vi "jog.vi"() -> ()   [LabVIEW 2018]
uses:
  <vilib>/MediaMongrels Ltd/WebSockets/WebSockets/WebSocket Client/WebSocket Client.lvclass
  D:/software_setup/National Instruments/LabVIEW 2018/vi.lib/MediaMongrels Ltd/WebSockets/WebSockets/WebSocket/WebSocket.lvclass
panel:
  out "GetJOGJointParams_acceleration":dbl[](array[numeric])
  out "GetJOGJointParams_velocity":dbl[](array[numeric])
  out "GetJOGCoordinateParams_acceleration":dbl[](array[numeric])
  out "GetJOGCoordinateParams_velocity":dbl[](array[numeric])
  out "accelerationRatio":i32
  out "velocityRatio":i32
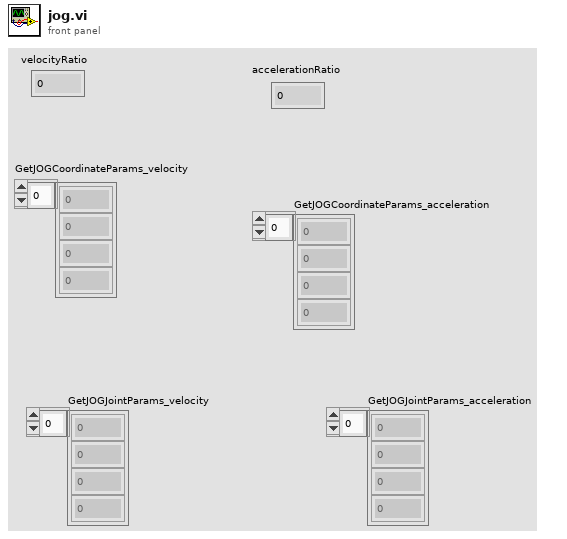
[diagram p1: front panel]
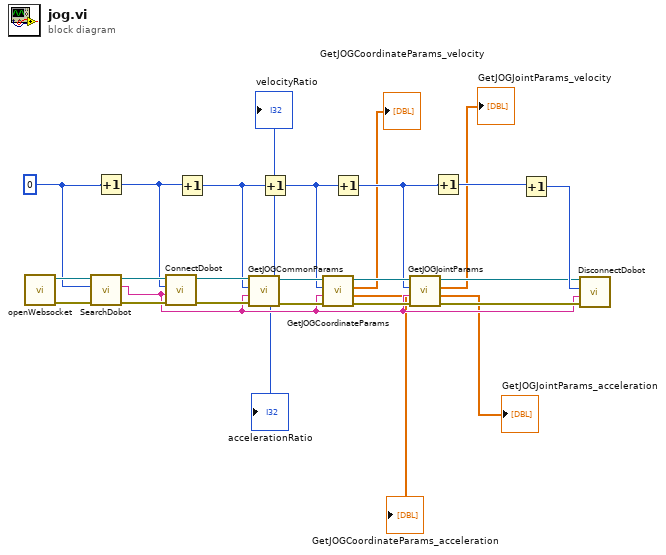
[diagram p0: block diagram]
diagram:
  w22 = 0 ("id")
  n1 = call <vilib>:"openWebsocket.vi"() -> ("error out"=w24:errorcluster, "WebSocket Client out"=w26:refnum<class "WebSocket Client.lvclass">)  [unwired: 10 in]
  n2 = call <vilib>:"SearchDobot.vi"("error in (no error)"=w24, "id"=w22, "WebSocket in"=w26) -> ("error out"=w23:errorcluster, "portName"=w7:string, "WebSocket out"=w25:refnum<class "WebSocket Client.lvclass">)  [unwired: 6 in]
  n3 = Increment(x=w22) -> (x+1=w21:i32)
  n4 = call <vilib>:"ConnectDobot.vi"("error in (no error)"=w23, "portName"=w7, "id"=w21, "WebSocket in"=w25) -> ("error out"=w14:errorcluster, "WebSocket out"=w18:refnum<class "WebSocket Client.lvclass">)  [unwired: 5 in, 1 out]
  n5 = Increment(x=w21) -> (x+1=w10:i32)
  n6 = call <vilib>:"GetJOGCommonParams.vi"("error in (no error)"=w14, "portName"=w7, "id"=w10, "WebSocket in"=w18) -> ("error out"=w13:errorcluster, "accelerationRatio"=→"accelerationRatio":i32, "velocityRatio"=→"velocityRatio":i32, "WebSocket out"=w17:refnum<class "WebSocket Client.lvclass">)  [unwired: 4 in]
  n7 = Increment(x=w10) -> (x+1=w9:i32)
  n8 = call <vilib>:"GetJOGCoordinateParams.vi"("error in (no error)"=w13, "portName"=w7, "id"=w9, "WebSocket in"=w17) -> ("error out"=w12:errorcluster, "acceleration"=→"GetJOGCoordinateParams_acceleration":dbl[], "velocity"=→"GetJOGCoordinateParams_velocity":dbl[], "WebSocket out"=w16:refnum<class "WebSocket Client.lvclass">)  [unwired: 4 in]
  n9 = Increment(x=w9) -> (x+1=w8:i32)
  n10 = call <vilib>:"GetJOGJointParams.vi"("error in (no error)"=w12, "portName"=w7, "id"=w8, "WebSocket in"=w16) -> ("error out"=w11:errorcluster, "acceleration"=→"GetJOGJointParams_acceleration":dbl[], "velocity"=→"GetJOGJointParams_velocity":dbl[], "WebSocket out"=w15:refnum<class "WebSocket Client.lvclass">)  [unwired: 4 in]
  n11 = Increment(x=w8) -> (x+1=w19:i32)
  n12 = Increment(x=w19) -> (x+1=w20:i32)
  n13 = call <vilib>:"DisconnectDobot.vi"("error in (no error)"=w11, "portName"=w7, "id"=w20, "WebSocket in"=w15) -> ()  [unwired: 5 in, 3 out]
